vi "timepulse_Cam_4.vi"(2 "de quantos segundos":i16=1) -> (1 "PULSO":bool)   [LabVIEW 2012]
panel:
  in  "Case Constant\n(See Context Help)":bool
  out "x+y":u32
  out "double precision float":dbl format="%#_10f"
  out "TIME ANTERIOR":u32
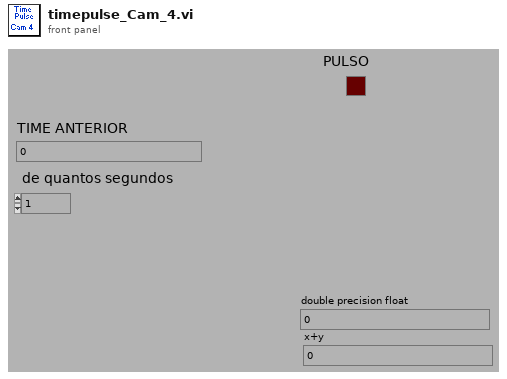
[diagram p1: front panel]
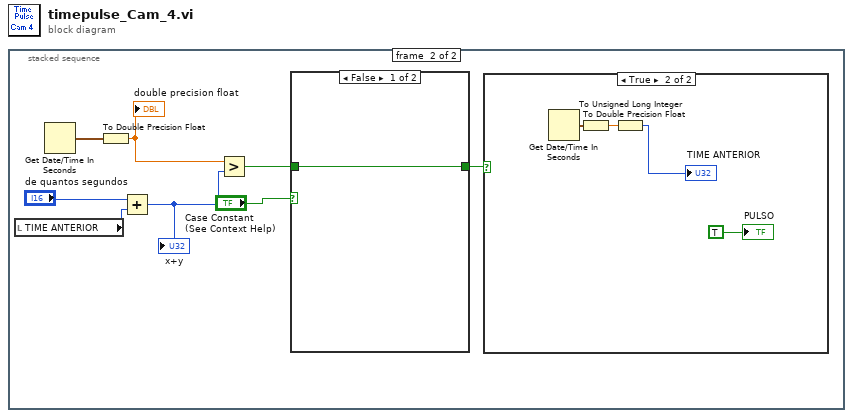
[diagram p0: block diagram]
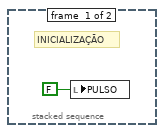
[diagram p2: hidden frame]
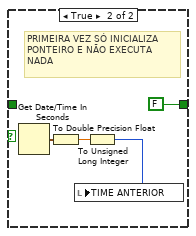
[diagram p3: hidden frame]
diagram:
  n1 = stacked-sequence {
    frame #0 {
      # "INICIALIZAÇÃO"
      n2 = local write "PULSO"(FALSE ("PULSO")) -> ()
    }
    frame #1 {
      n3 = local read "TIME ANTERIOR"() -> (w5:u32)
      n4 = Get Date/Time In Seconds() -> (seconds since 1Jan1904=w7:timestamp)
      n5 = To Double Precision Float(number=w7) -> (double precision float=w3:dbl)
      "double precision float" <- w3
      n6 = Add(x="de quantos segundos", y=w5) -> (x+y=w4:u32)
      "x+y" <- w4
      n7 = Greater?(x=w3, y=w4) -> (0:w9:bool)
      n8 = case shown="False" "Case Constant\n(See Context Help)" {
        tunnel: w9 -> [w10 _]
        tunnel: [w10 FALSE] -> w8
        frame False {
        }
        frame True {
          # "PRIMEIRA VEZ SÓ INICIALIZA\nPONTEIRO E NÃO EXECUTA\nNADA"
          n9 = Get Date/Time In Seconds() -> (seconds since 1Jan1904=w12:timestamp)
          n10 = To Double Precision Float(number=w12) -> (double precision float=w11:dbl)
          n11 = To Unsigned Long Integer(number=w11) -> (unsigned 32bit integer=w14:u32)
          n12 = local write "TIME ANTERIOR"(w14) -> ()
        }
      }
      n13 = case shown="True" w8 {
        frame False {
        }
        frame True {
          n14 = Get Date/Time In Seconds() -> (seconds since 1Jan1904=w16:timestamp)
          n15 = To Double Precision Float(number=w16) -> (double precision float=w15:dbl)
          n16 = To Unsigned Long Integer(number=w15) -> (unsigned 32bit integer=→"TIME ANTERIOR":u32)
          "PULSO" <- TRUE ("PULSO")
        }
      }
    }
  }
